vi "CvrtCell2Data.vi"(8 "error in (no error)":errorcluster, 9 "ge_HdrNames":T1, 10 "Item Name":string, 11 "Frequency in":refnum<class "Frequency.lvclass">) -> (0 "error out":errorcluster, 3 "Frequency out":refnum<class "Frequency.lvclass">)   [LabVIEW 2018, in "Measurement Channels.lvlib" / "Frequency.lvclass"]
uses:
  Frequency.lvclass
  Common/Controls/HeaderNames.ctl
  Frequency.lvclass/Frequency.ctl
  SubVIs Table/Custom Ctls Table/ge_ColType.ctl
  Class Voltage/Voltage.lvclass
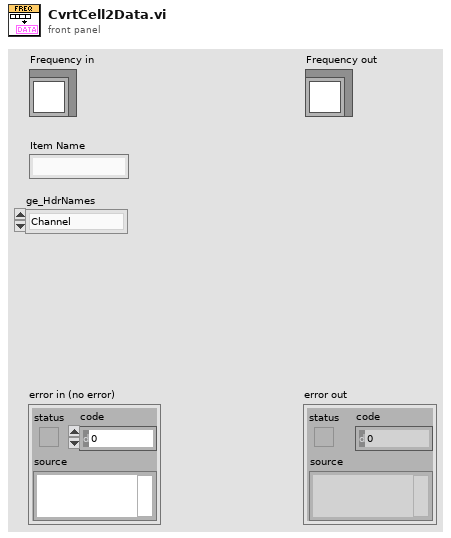
[diagram p1: front panel]
types:
  T1 = typedef "HeaderNames.ctl" = enum16{"Channel", "Device", "Spacer", "Description", "MB", "Range", "Terminal", "Coupling", "Thresh (V)", "Pulse/Rev", "Slope", "Min EU", "Min RPM", "mV/EU", "Iex", "Temp Units", "Type", "CJC Src", "CJC Val", "Ro", "Wire Cfg", "Strain Mode", "Vex", "Bridge Type", "GF", "Gauge Res", "Poisson", "Lead Res", "Init Strain", "GAF", "Scale", "Offset", "Unit (EU)", "dB?", "dB Ref", "Cal Mag", "Cal Units", "Max Temp", "Min Temp", "Max Strain", "Min Strain"}
  T2 = typedef "ge_ColType.ctl" = enum16{"Volts", "Amps", "Ohms", "TermCfg", "WireCfg", "Coup", "Slope", "Iex", "CalUnits", "ThrmUnits", "ThrmType", "CJCSrc", "BrdgType", "Strn Mode", "RTDType"}
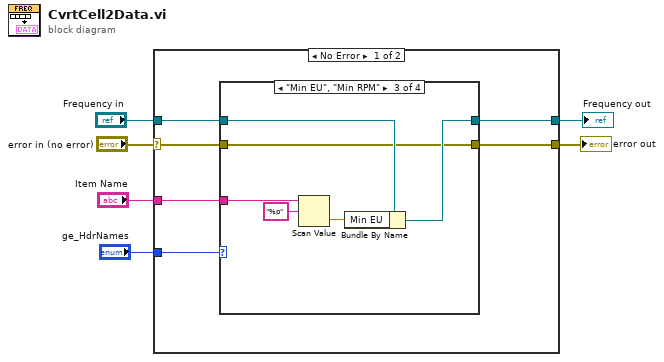
[diagram p0: block diagram]
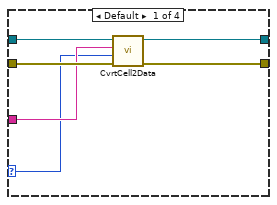
[diagram p2: hidden frame]
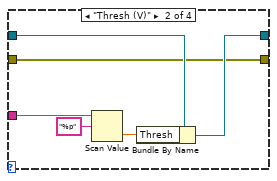
[diagram p3: hidden frame]
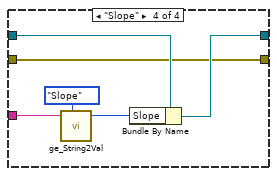
[diagram p4: hidden frame]
diagram:
  n1 = case shown="No Error" "error in (no error)" {
    selector: "error in (no error)" -> [w8 w37]
    tunnel: "Frequency in" -> [w12 w38]
    tunnel: [w11 w38] -> w5
    tunnel: [w7 w37] -> w4
    tunnel: "Item Name" -> [w10 _]
    tunnel: "ge_HdrNames" -> [w9 _]
    frame No Error {
      n2 = case shown="\"Min EU\", \"Min RPM\"" w9 {
        selector: w9 -> [w13 _ _ _]
        tunnel: w10 -> [w14 w19 w26 w33]
        tunnel: w12 -> [w18 w23 w29 w36]
        tunnel: [w17 w24 w30 w35] -> w11
        tunnel: w8 -> [w16 w22 w28 w31]
        tunnel: [w15 w22 w28 w31] -> w7
        frame Default {
          n3 = call-parent "CvrtCell2Data.vi"("error in"=w16, "ge_HdrNames"=w13, "Item Name"=w14, "Voltage In"=w18) -> ("error out"=w15:errorcluster, "Voltage Out"=w17:refnum<class "Frequency.lvclass">)  [unwired: 6 in]
        }
        frame "Thresh (V)" {
          n4 = Scan Value(string=w19, format string="%p") -> (value=w20:dbl)  [unwired: 1 in, 1 out]
          n5 = Bundle By Name(cluster=w23, "Thresh"=w20) -> (w24:refnum<class "Frequency.lvclass">)
        }
        frame "Min EU", "Min RPM" {
          n6 = Scan Value(string=w26, format string="%p") -> (value=w25:dbl)  [unwired: 1 in, 1 out]
          n7 = Bundle By Name(cluster=w29, "Min EU"=w25) -> (w30:refnum<class "Frequency.lvclass">)
        }
        frame "Slope" {
          n8 = call "ge_String2Val.vi"("String"=w33, "ColType"=ge_ColType."Slope") -> ("Value"=w32:u16)  [unwired: 4 in, 1 out]
          n9 = Bundle By Name(cluster=w36, "Slope"=w32) -> (w35:refnum<class "Frequency.lvclass">)
        }
      }
    }
    frame Error {
    }
  }
  "error out" <- w4
  "Frequency out" <- w5
